vi "Get Acyclic Buffer ID.vi"(8 "error in":errorcluster, 11 "acyclic frame trigger in":T1 format="%.0x") -> (0 "error out":errorcluster, 2 "acyclic buffer ID":string, 3 "acyclic frame trigger out":T1 format="%.0x")   [LabVIEW 2020, in "Ballard MIL-STD-1553 Scripting.lvlib"]
uses:
  Ballard MIL-STD-1553 Scripting.lvlib
  <vilib>/NI VeriStand/Custom Device API/Custom Device Item Ref.ctl
  Constants.vi
  <vilib>/NI VeriStand/Custom Device API/Get Item Property (String).vi
  <vilib>/NI VeriStand/Custom Device API/Custom Device API.lvlib
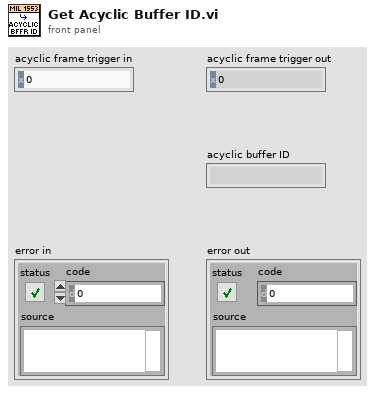
[diagram p1: front panel]
types:
  T1 = typedef "Custom Device API.lvlib/Custom Device Item Ref.ctl" = u64
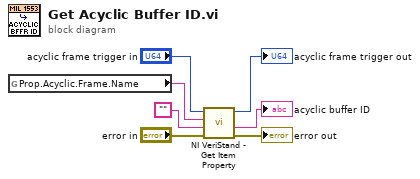
[diagram p0: block diagram]
diagram:
  n1 = global read "Constants.vi" "Prop.Acyclic.Frame.Name"() -> (w7:string)
  n2 = call-poly <vilib>:"NI VeriStand - Get Item Property.vi"("error in (no error)"="error in", "Default Value"="", "Property Name"=w7, "Item Ref in"="acyclic frame trigger in") -> ("error out"=→"error out":errorcluster, "Value"=→"acyclic buffer ID":string, "Item Ref out"=→"acyclic frame trigger out":T1)  [unwired: 4 in, 1 out]
